vi "TLB Native Dynamic Events ver 0.04d.vi"() -> ()   [LabVIEW 2018]
uses:
  Labview Training Phase 2/Enum Controls/States for Action Engine.ctl
  Type def/TLB event states.ctl
  Type def/TLB MHL States.ctl
  <vilib>/Studica/Studica Toolkit/Background/I2C Channel.ctl
  <vilib>/Studica/Studica Toolkit/NavX/NavX.lvlib
  <vilib>/myRIO/Common/Instrument Driver Framework/myRIO v1.0/AI/typedefs/AI Channels Enum.ctl
  <vilib>/myRIO/Common/Instrument Driver Framework/myRIO v1.0/AI/typedefs/AI Channels List.ctl
  <vilib>/Studica/Studica Toolkit/Background/Mxp Selection.ctl
  <vilib>/ptbypt/NI_PtbyPt.lvlib
panel:
  out "Distance":T1
  in  "Return to IDLE":bool
  out "Sharp IR Distance":dbl
  out "Sharp IR Distance 2":dbl
  out "CM":fxp<+,64,16>
  out "Ultrasonic sensor":dbl format="%0.2f"
  out "Waveform Chart 3":dbl(graph)
  out "NavX Info Out":T3
  out "LinearAcceleration":T4
  out "Displacement":T5
  out "YRPHfH":T6
  in  "xTargetSpeed":dbl
  in  "yTargetSpeed":dbl
  in  "wTargetSpeed":dbl
  out "Speed":T7
  in  "Reset Encoder 0":bool
  out "Action Queue Items":i32
  out "State Logic Queue Items":i32
  out "Action Queues items":string[](array[string])=["Hardware reset", "Software reset", ""]
  out "State logic":T8=enum."Task 2"
  out "Action State":string
  in  "Tasks Selector":string(combo)="Task 2"
  in  "Stop Queue":bool
  in  "Start Task":bool
  # "Test Programme written by Calvin Loke    Dated: 28 Aug 2019\nTest Programme revised by Dr Alex See   Dated 30 Aug 2019\n\nProgramme version:   TLB Native Dynamic Events ver 0.04b.vi"
  # "System Health Status Update"
  # "Sequence of Actions"
  # "Continuous (Repeated)"
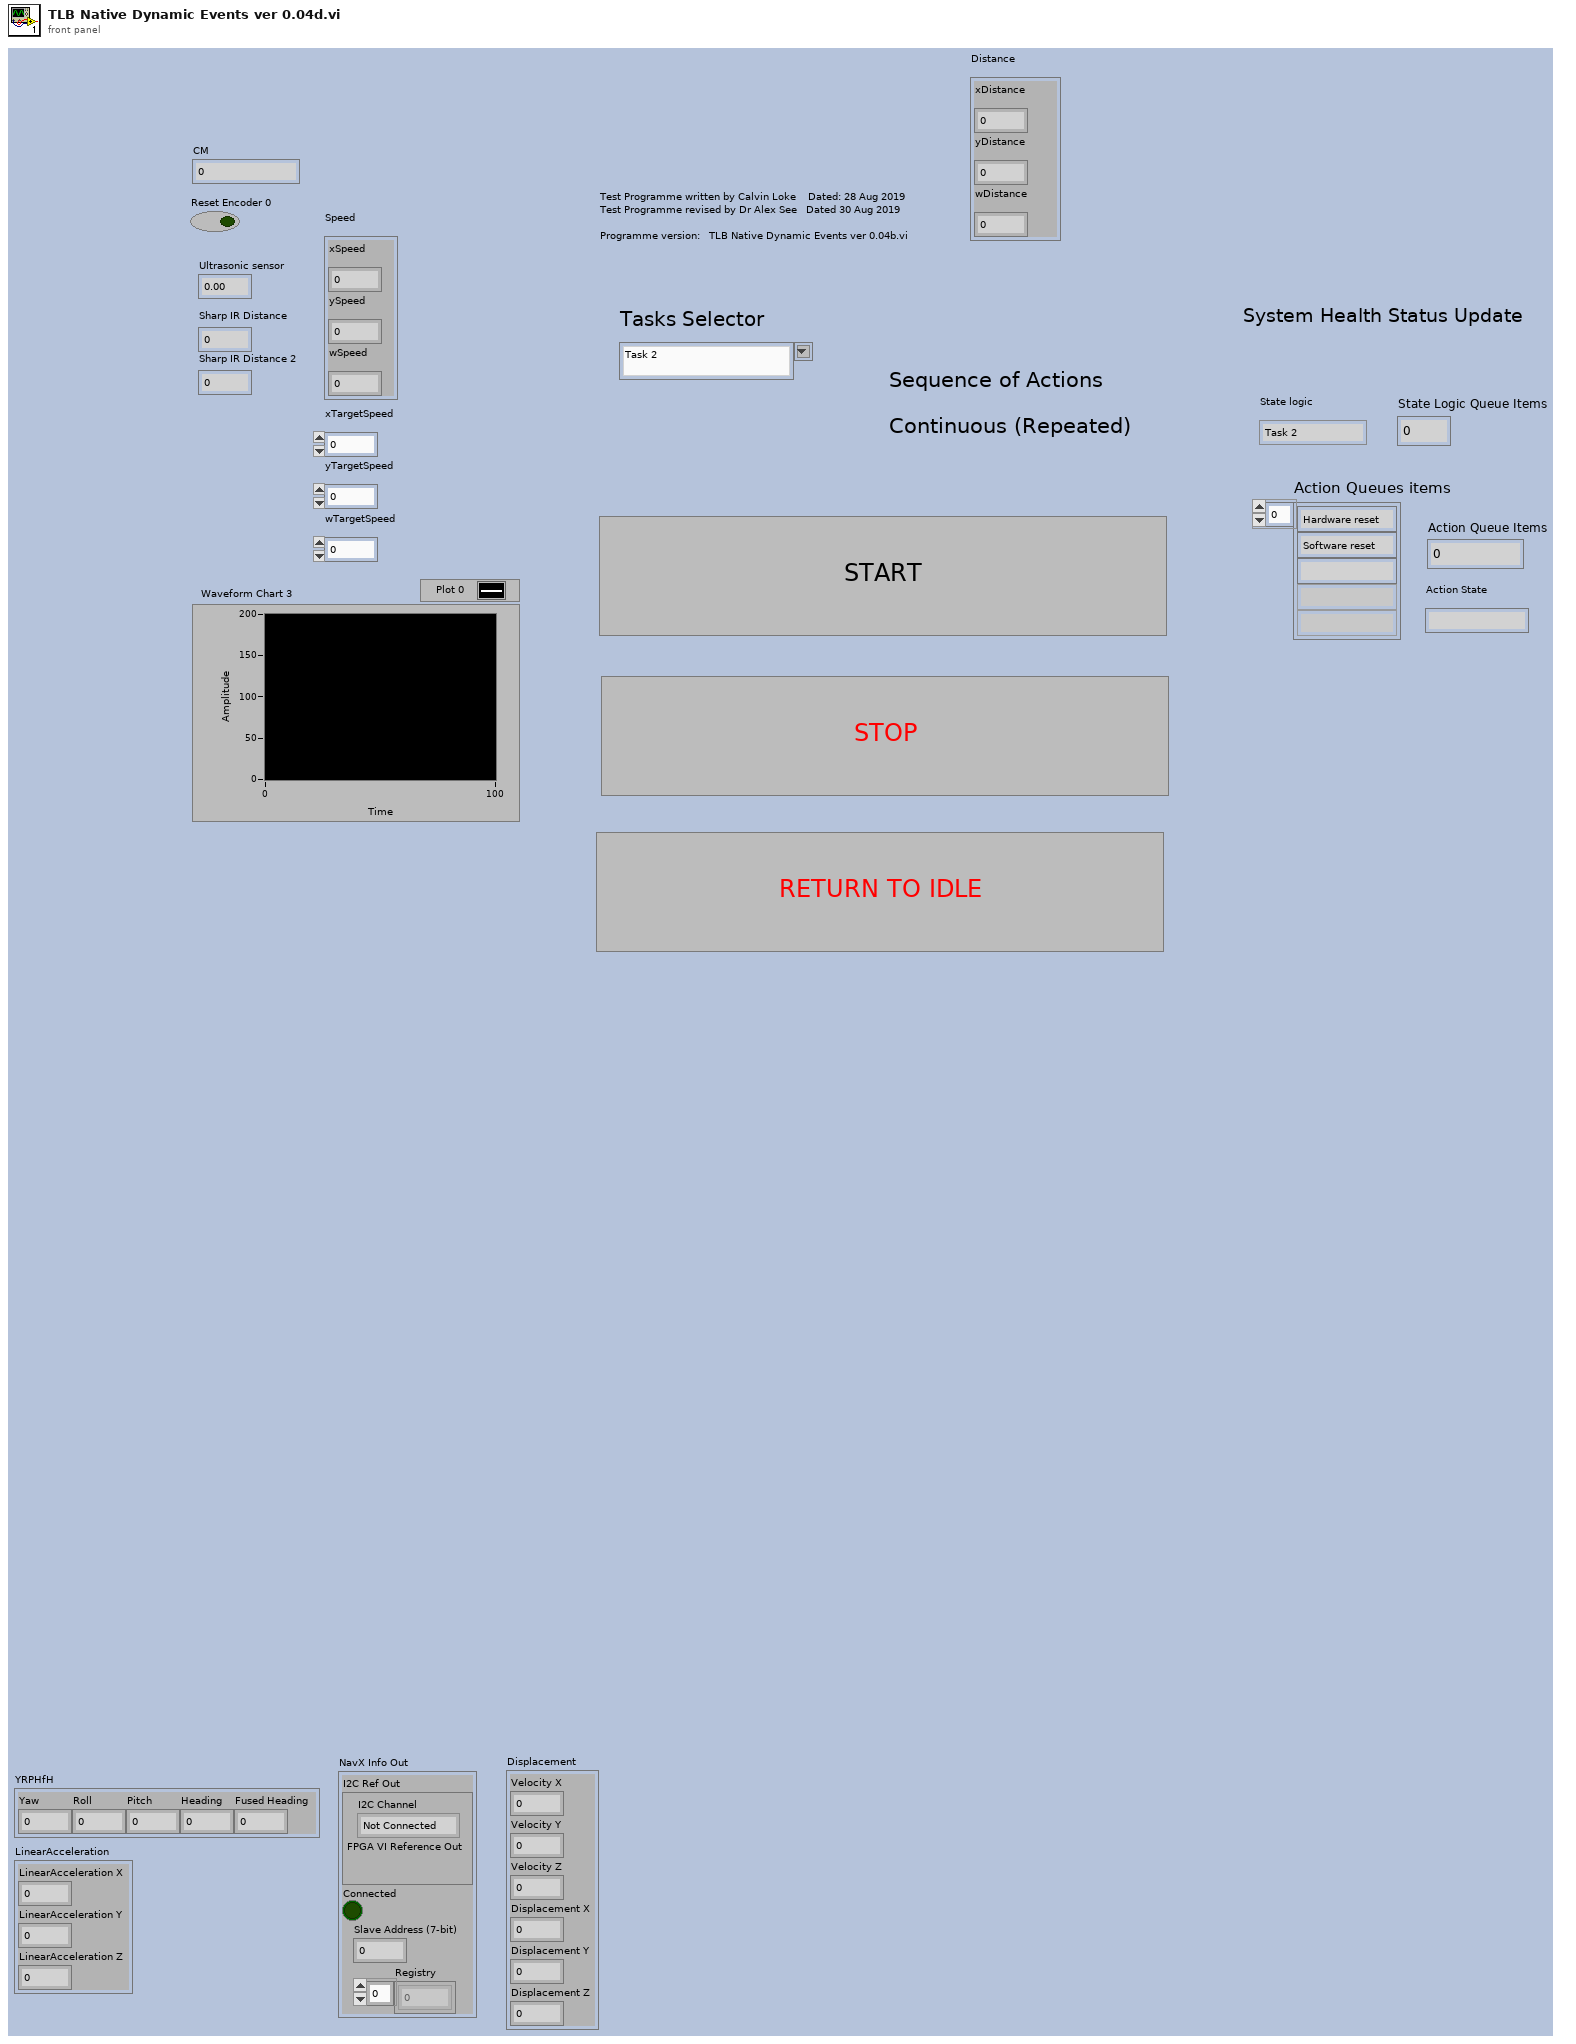
[diagram p1: front panel]
types:
  T1 = cluster{"xDistance":dbl, "yDistance":dbl, "wDistance":dbl}
  T2 = typedef "I2C Channel.ctl" = enum16{"Not Connected", "A", "B"}
  T3 = cluster{"I2C Ref Out":cluster{"I2C Channel":T2, "FPGA VI Reference Out":refnum<k20>}, "Connected":bool, "Slave Address (7-bit)":u8, "Registry":u8[]}
  T4 = cluster{"LinearAcceleration X":dbl, "LinearAcceleration Y":dbl, "LinearAcceleration Z":dbl}
  T5 = cluster{"Velocity X":dbl, "Velocity Y":dbl, "Velocity Z":dbl, "Displacement X":dbl, "Displacement Y":dbl, "Displacement Z":dbl}
  T6 = cluster{"Yaw":dbl, "Roll":dbl, "Pitch":dbl, "Heading":dbl, "Fused Heading":dbl}
  T7 = cluster{"xSpeed":dbl, "ySpeed":dbl, "wSpeed":dbl}
  T8 = typedef "TLB MHL States.ctl" = enum16{"None", "Startup", "Idle", "Processing", "Shutdown", "Reset", "Task 1", "Task 2", "Task 3", "Task 4", "Task 4a", "Task 4b", "Task 4c", "Task 4d", "Task 4e", "Task 4f", "Task 4g", "Task 4h", "Acquire image", "Wall follow mode", "Autodrive", "Autodrive a"}
  T9 = typedef "States for Action Engine.ctl" = enum16{"Initialize", "Write", "Read"}
  T10 = typedef "TLB event states.ctl" = enum16{"Start Sequence", "Exit", "Start Task 1", "Start Task 2", "Start Task 3", "Start Task 4", "Camera vision", "Wall follow mode", "Idle", "Start Drive Straight"}
  T11 = typedef "Mxp Selection.ctl" = enum16{"MXP A", "MXP B"}
  T12 = typedef "TLB event states.ctl" = enum16{"Start Sequence", "Exit", "Task 1", "Task 2", "Idle"}
  T13 = typedef "AI Channels List.ctl" = T14[]
  T14 = typedef "AI Channels Enum.ctl" = enum16{"Not Connected", "AudioIn/Left", "AudioIn/Right", "C/AI0", "C/AI1", "A/AI0", "A/AI1", "A/AI2", "A/AI3", "A/AI4", "A/AI5", "A/AI6", "A/AI7", "B/AI0", "B/AI1", "B/AI2", "B/AI3", "B/AI4", "B/AI5", "B/AI6", "B/AI7", "AI/AI0", "AI/AI1", "AI/AI2", "AI/AI3", "A/AI0 (DIFF)", "A/AI1 (DIFF)", "A/AI2 (DIFF)", "A/AI3 (DIFF)", "B/AI0 (DIFF)", "B/AI1 (DIFF)", "B/AI2 (DIFF)", "B/AI3 (DIFF)"}
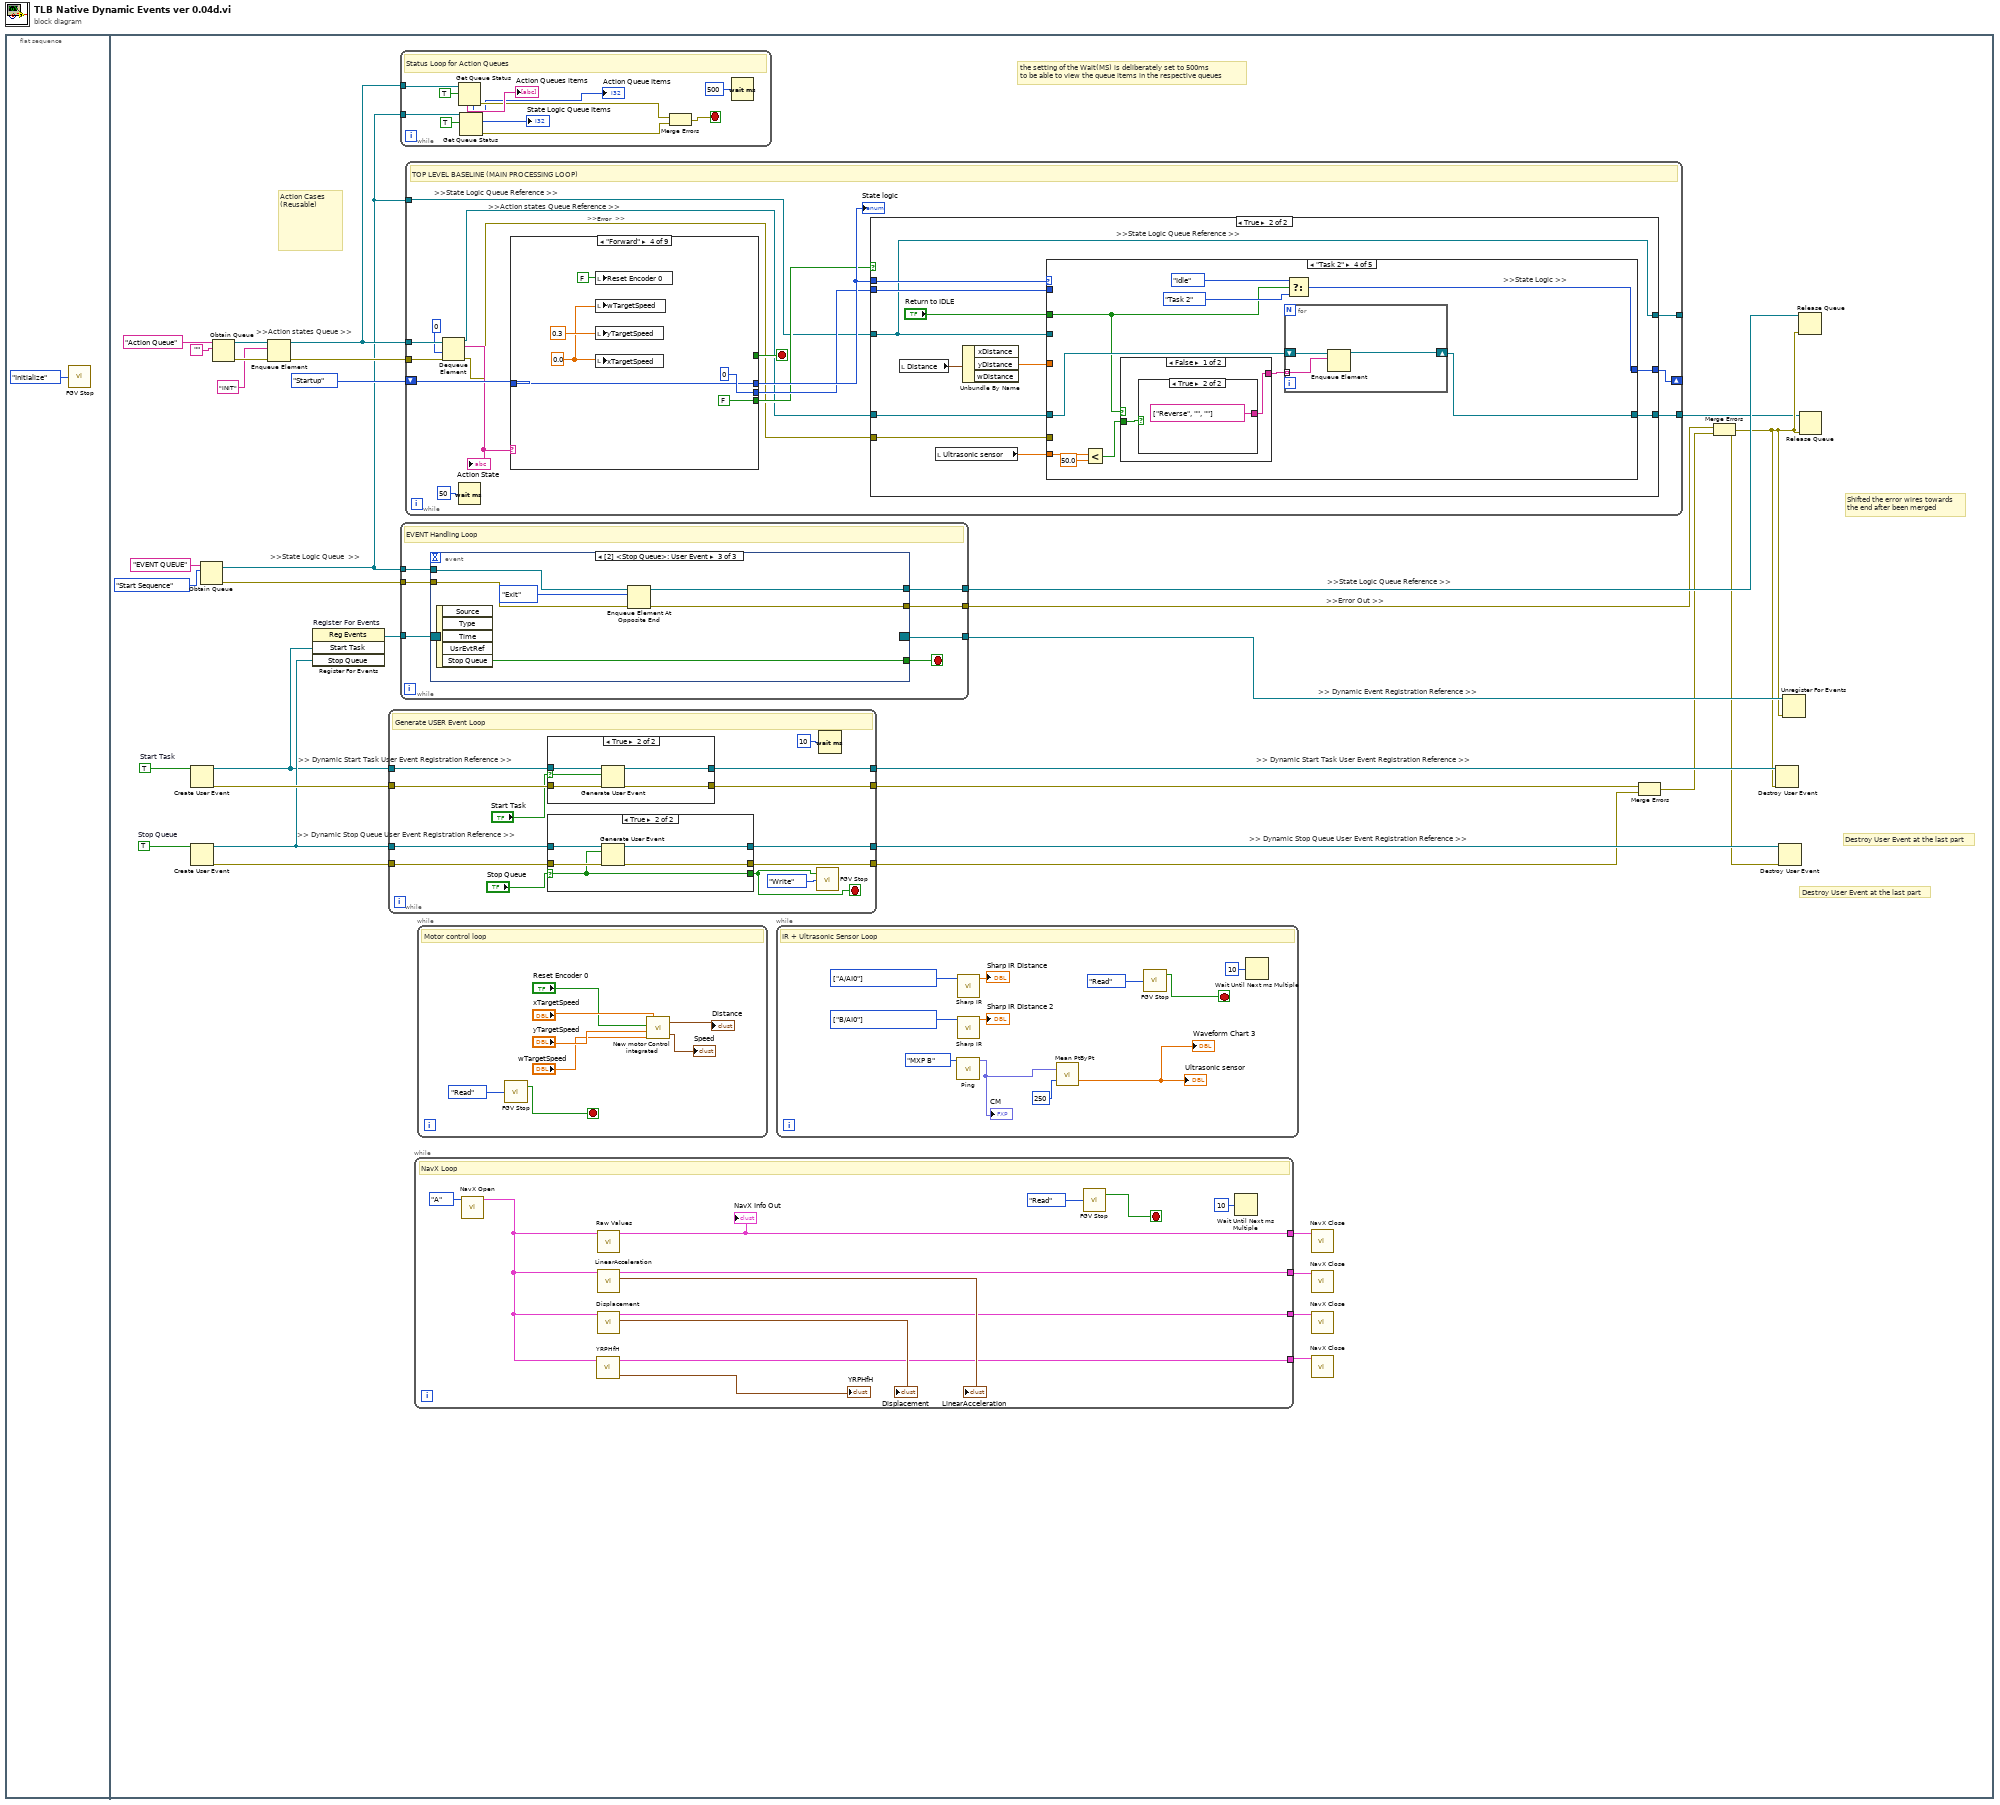
[diagram p0: block diagram]
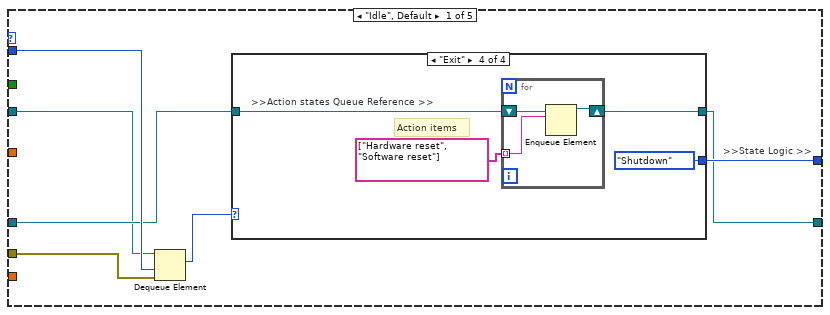
[diagram p3: hidden frame]
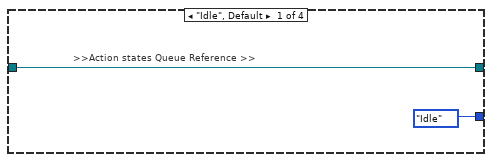
[diagram p4: hidden frame]
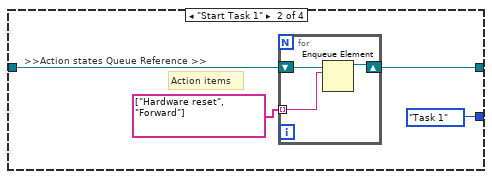
[diagram p5: hidden frame]
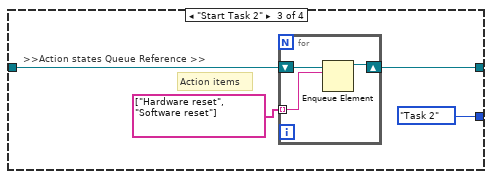
[diagram p6: hidden frame]
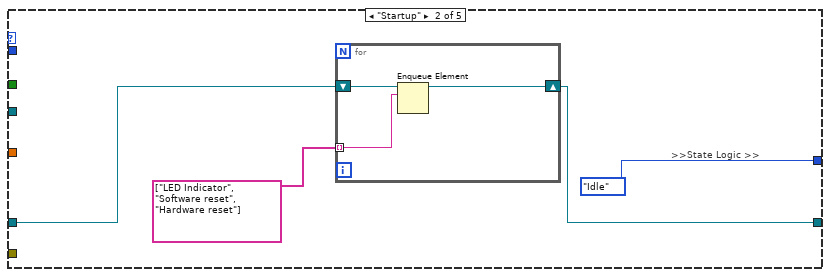
[diagram p7: hidden frame]
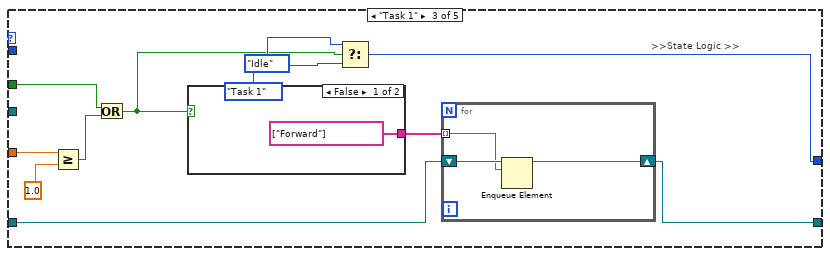
[diagram p8: hidden frame]
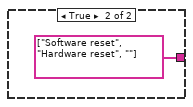
[diagram p9: hidden frame]
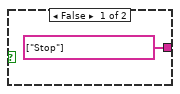
[diagram p10: hidden frame]
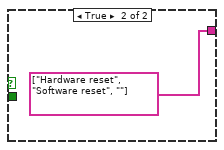
[diagram p11: hidden frame]
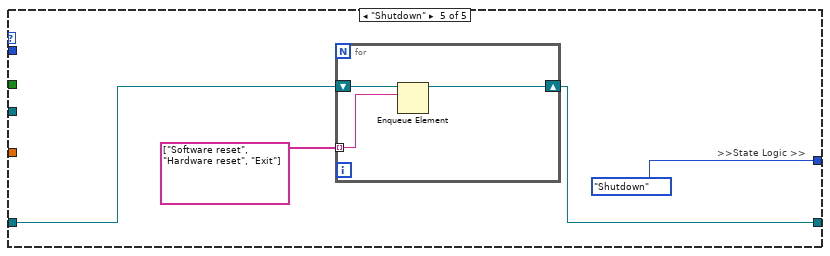
[diagram p12: hidden frame]
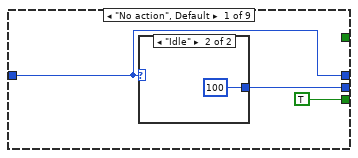
[diagram p13: hidden frame]
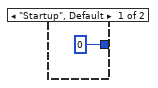
[diagram p14: hidden frame]
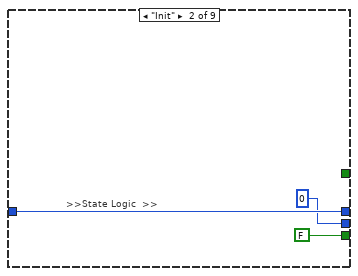
[diagram p15: hidden frame]
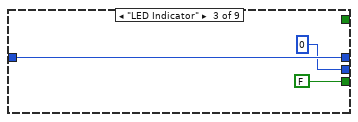
[diagram p16: hidden frame]
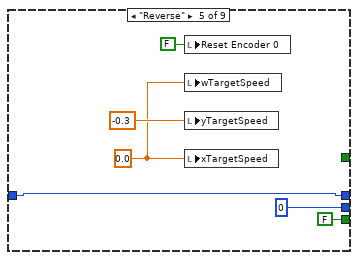
[diagram p17: hidden frame]
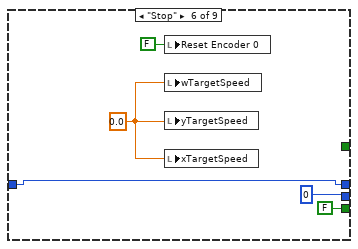
[diagram p18: hidden frame]
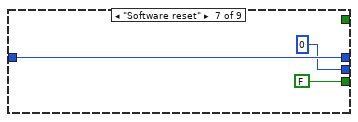
[diagram p19: hidden frame]
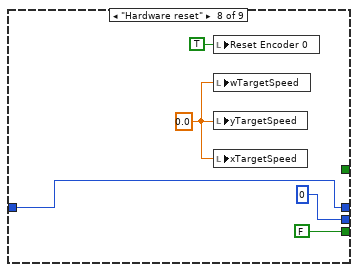
[diagram p20: hidden frame]
diagram:
  n1 = flat-sequence {
    frame #0 {
      n2 = call "FGV Stop.vi"("Init/Read/Write State"=States_for_Action_Engine."Initialize") -> ()  [unwired: 2 in, 2 out]
    }
    frame #1 {
      w34 = TRUE  # Stop Queue
      w33 = TRUE  # Start Task
      # "the setting of the Wait(MS) is deliberately set to 500ms\nto be able to view the queue items in the respective queues"
      # "Action Cases\n(Reusable)"
      # ">>Error Out >>"
      # ">> Dynamic Stop Queue User Event Registration Reference >>"
      # ">> Dynamic Start Task User Event Registration Reference >>"
      # ">> Dynamic Stop Queue User Event Registration Reference >>"
      # ">> Dynamic Start Task User Event Registration Reference >>"
      # ">> Dynamic Event Registration Reference >>"
      # ">>Action states Queue >>"
      # ">>State Logic Queue  >>"
      # ">>State Logic Queue Reference >>"
      # "Destroy User Event at the last part"
      # "Destroy User Event at the last part"
      # "Shifted the error wires towards\nthe end after been merged"
      n3 = Create User Event(user event datatype=w33) -> (user event=w25:refnum<user-event>, error out=w30:errorcluster)  [unwired: 1 in]
      n4 = Create User Event(user event datatype=w34) -> (user event=w26:refnum<user-event>, error out=w29:errorcluster)  [unwired: 1 in]
      n5 = Obtain Queue(name (unnamed)="EVENT QUEUE", element data type=TLB_event_states."Start Sequence" ("Enum")) -> (queue out=w9:refnum<queue>, error out=w15:errorcluster)  [unwired: 3 in, 1 out]
      n6 = Obtain Queue(name (unnamed)="Action Queue", element data type="") -> (queue out=w18:refnum<queue>, error out=w14:errorcluster)  [unwired: 3 in, 1 out]
      n7 = Enqueue Element(queue=w18, element="INIT", error in (no error)=w14) -> (queue out=w10:refnum<queue>, error out=w13:errorcluster)  [unwired: 1 in, 1 out]
      n8 = register-events "Register For Events"(w25, w26) -> (reference out=w24:refnum<event-registration>)  [unwired: 2 in, 1 out]
      n9 = while {
        tunnel: w25 -> [w265]
        tunnel: w26 -> [w264]
        tunnel: [w263] -> w32
        tunnel: [w262] -> w31
        tunnel: w30 -> [w261]
        tunnel: [w260] -> w28
        tunnel: w29 -> [w259]
        tunnel: [w258] -> w27
        stop <- w254 stop-if-true
        # "Generate USER Event Loop"
        n10 = case shown="True" "Start Task" {
          selector: "Start Task" -> [_ w277]
          tunnel: w265 -> [w276 w281]
          tunnel: [w276 w280] -> w262
          tunnel: w261 -> [w275 w279]
          tunnel: [w275 w278] -> w260
          frame False {
          }
          frame True {
            n11 = Generate User Event(user event=w281, event data cluster=w277, error in=w279) -> (user event out=w280:refnum<user-event>, error out=w278:errorcluster)  [unwired: 1 in]
          }
        }
        n12 = case shown="True" "Stop Queue" {
          selector: "Stop Queue" -> [_ w270]
          tunnel: w264 -> [w269 w274]
          tunnel: [w269 w273] -> w263
          tunnel: w259 -> [w268 w272]
          tunnel: [w268 w271] -> w258
          tunnel: [FALSE w270] -> w254
          frame False {
          }
          frame True {
            n13 = Generate User Event(user event=w274, event data cluster=w270, error in=w272) -> (user event out=w273:refnum<user-event>, error out=w271:errorcluster)  [unwired: 1 in]
          }
        }
        n14 = call "FGV Stop.vi"("Init/Read/Write State"=States_for_Action_Engine."Write", "Input Node"=w254) -> ()  [unwired: 1 in, 2 out]
        n15 = Wait (ms)(milliseconds to wait=u32 10) -> ()  [unwired: 1 out]
      }
      n16 = while {
        tunnel: w10 -> [w74]
        tunnel: w9 -> [w71]
        stop <- w68 stop-if-true
        # "Status Loop for Action Queues"
        n17 = Get Queue Status(queue=w74, return elements? (F)=TRUE) -> (error out=w70:errorcluster, # elements in queue=→"Action Queue Items":i32, elements=→"Action Queues items":string[])  [unwired: 1 in, 5 out]
        n18 = Get Queue Status(queue=w71, return elements? (F)=TRUE) -> (# pending remove=→"State Logic Queue Items":i32, error out=w69:errorcluster)  [unwired: 1 in, 6 out]
        n19 = Merge Errors(w70, w69) -> (w68:errorcluster)
        n20 = Wait (ms)(milliseconds to wait=u32 500) -> ()  [unwired: 1 out]
      }
      n21 = while {
        tunnel: w24 -> [w231]
        tunnel: [w230] -> w23
        tunnel: w9 -> [w228]
        tunnel: [w227] -> w22
        tunnel: w15 -> [w226]
        tunnel: [w225] -> w12
        stop <- w229 stop-if-true
        # "EVENT Handling Loop"
        n22 = event shown="[2] <Stop Queue>: User Event" {
          selector: w231 -> [_ _ _]
          dyn-events: [_ _ _] -> w230
          timeout: _ -> [_ _ _]
          tunnel: [FALSE FALSE w253] -> w229
          tunnel: w228 -> [w236 w243 w251]
          tunnel: [w235 w242 w252] -> w227
          tunnel: w226 -> [w233 w239 w249]
          tunnel: [w232 w238 w248] -> w225
          event Timeout {
            n23 = event-data() -> ()  [unwired: 1 in, 3 out]
            n24 = Enqueue Element(queue=w236, element=TLB_event_states."Idle" ("Enum"), error in (no error)=w233) -> (queue out=w235:refnum<queue>, error out=w232:errorcluster)  [unwired: 1 in, 1 out]
          }
          event User Event {
            n25 = event-data() -> ()  [unwired: 1 in, 5 out]
            n26 = case shown="Default" "Tasks Selector" {
              tunnel: [TLB_event_states."Idle" ("Enum") TLB_event_states."Start Task 1" ("Enum") TLB_event_states."Task 2" ("Enum")] -> w240
              frame Default {
              }
              frame "Task 1" {
              }
              frame "Task 2" {
              }
            }
            n27 = Enqueue Element(queue=w243, element=w240, error in (no error)=w239) -> (queue out=w242:refnum<queue>, error out=w238:errorcluster)  [unwired: 1 in, 1 out]
          }
          event User Event {
            n28 = event-data() -> ("Stop Queue"=w253:bool)  [unwired: 1 in, 4 out]
            n29 = Enqueue Element At Opposite End(queue=w251, element=TLB_event_states."Exit" ("Enum"), error in (no error)=w249) -> (queue out=w252:refnum<queue>, error out=w248:errorcluster)  [unwired: 1 in, 1 out]
          }
        }
      }
      n30 = while {
        tunnel: w9 -> [w79]
        shift-right: [w84] -> _
        shift-left: TLB_MHL_States."Startup" ("Enum") -> [w91]
        tunnel: w10 -> [w89]
        tunnel: w13 -> [w87]
        tunnel: [w86] -> _
        tunnel: [w85] -> w7
        stop <- w82 stop-if-true
        # ">>Error  >>"
        # ">>Action states Queue Reference >>"
        # ">>State Logic Queue Reference >>"
        # "TOP LEVEL BASELINE (MAIN PROCESSING LOOP)"
        n31 = Dequeue Element(queue=w89, timeout in ms (-1)=0, error in (no error)=w87) -> (queue out=w78:refnum<queue>, element=w88:string, error out=w77:errorcluster)  [unwired: 1 out]
        "Action State" <- w88
        n32 = Wait (ms)(milliseconds to wait=u32 50) -> ()  [unwired: 1 out]
        n33 = case shown="\"Forward\"" w88 {
          tunnel: [w187 w192 w195 w200 w206 w211 w215 w220 TLB_MHL_States."Shutdown" ("Enum")] -> w90
          tunnel: w91 -> [w187 w192 w195 w200 w206 w211 w215 w220 _]
          tunnel: [w186 0 0 0 0 0 0 0 0] -> w83
          tunnel: [_ _ _ _ _ _ _ _ TRUE] -> w82
          tunnel: [TRUE FALSE FALSE FALSE FALSE FALSE FALSE FALSE FALSE] -> w81
          frame "No action", Default {
            n34 = case shown="\"Idle\"" w187 {
              tunnel: [0 100] -> w186
              frame "Startup", Default {
              }
              frame "Idle" {
              }
            }
          }
          frame "Init" {
            # ">>State Logic  >>"
          }
          frame "LED Indicator" {
          }
          frame "Forward" {
            w196 = 0.0
            n35 = local write "Reset Encoder 0"(FALSE ("Reset Encoder 0")) -> ()
            n36 = local write "wTargetSpeed"(w196) -> ()
            n37 = local write "yTargetSpeed"(0.3 ("yTargetSpeed")) -> ()
            n38 = local write "xTargetSpeed"(w196) -> ()
          }
          frame "Reverse" {
            w202 = 0.0
            n39 = local write "Reset Encoder 0"(FALSE ("Reset Encoder 0")) -> ()
            n40 = local write "wTargetSpeed"(w202) -> ()
            n41 = local write "yTargetSpeed"(-0.3 ("yTargetSpeed")) -> ()
            n42 = local write "xTargetSpeed"(w202) -> ()
          }
          frame "Stop" {
            w208 = 0.0
            n43 = local write "Reset Encoder 0"(FALSE ("Reset Encoder 0")) -> ()
            n44 = local write "wTargetSpeed"(w208) -> ()
            n45 = local write "yTargetSpeed"(w208) -> ()
            n46 = local write "xTargetSpeed"(w208) -> ()
          }
          frame "Software reset" {
          }
          frame "Hardware reset" {
            w216 = 0.0
            n47 = local write "Reset Encoder 0"(TRUE ("Reset Encoder 0")) -> ()
            n48 = local write "wTargetSpeed"(w216) -> ()
            n49 = local write "yTargetSpeed"(w216) -> ()
            n50 = local write "xTargetSpeed"(w216) -> ()
          }
          frame "Exit" {
          }
        }
        "State logic" <- w90
        n51 = case shown="True" w81 {
          tunnel: w90 -> [w94 w106]
          tunnel: w79 -> [w95 w100]
          tunnel: w78 -> [w93 w105]
          tunnel: [w95 w100] -> w86
          tunnel: [w93 w104] -> w85
          tunnel: [w94 w103] -> w84
          tunnel: w77 -> [_ w102]
          tunnel: w83 -> [_ w101]
          frame False {
          }
          frame True {
            # ">>State Logic Queue Reference >>"
            n52 = local read "Distance"() -> (w98:T1)
            n53 = local read "Ultrasonic sensor"() -> (w96:dbl)
            n54 = Unbundle By Name(w98) -> ("yDistance"=w97:dbl)  [unwired: 2 out]
            n55 = case shown="\"Task 2\"" w106 {
              tunnel: w100 -> [w107 _ _ _ _]
              tunnel: w105 -> [w109 w138 w150 w165 w179]
              tunnel: [w108 w137 w149 w166 w178] -> w104
              tunnel: [w112 TLB_MHL_States."Idle" ("Enum") w152 w167 TLB_MHL_States."Shutdown" ("Enum")] -> w103
              tunnel: w102 -> [w110 _ _ _ _]
              tunnel: w101 -> [w111 _ _ _ _]
              tunnel: "Return to IDLE" -> [_ _ w147 w162 _]
              tunnel: w97 -> [_ _ w146 _ _]
              tunnel: w96 -> [_ _ _ w164 _]
              frame "Idle", Default {
                # ">>State Logic >>"
                n56 = Dequeue Element(queue=w107, timeout in ms (-1)=w111, error in (no error)=w110) -> (element=w113:T10)  [unwired: 3 out]
                n57 = case shown="\"Exit\"" w113 {
                  tunnel: [TLB_MHL_States."Idle" ("Enum") TLB_MHL_States."Task 1" ("Enum") TLB_MHL_States."Task 2" ("Enum") TLB_MHL_States."Shutdown" ("Enum")] -> w112
                  tunnel: [w114 w118 w123 w130] -> w108
                  tunnel: w109 -> [w114 w116 w124 w131]
                  frame "Idle", Default {
                    # ">>Action states Queue Reference >>"
                  }
                  frame "Start Task 1" {
                    # ">>Action states Queue Reference >>"
                    # "Action items"
                    n58 = for {
                      shift-right: [w122] -> w118
                      shift-left: w116 -> [w121]
                      tunnel: string[] ["Hardware reset", "Forward"] -> [w120] mode=indexing
                      n59 = Enqueue Element(queue=w121, element=w120) -> (queue out=w122:refnum<queue>)  [unwired: 2 in, 2 out]
                    }
                  }
                  frame "Start Task 2" {
                    # ">>Action states Queue Reference >>"
                    # "Action items"
                    n60 = for {
                      shift-right: [w129] -> w123
                      shift-left: w124 -> [w128]
                      tunnel: string[] ["Hardware reset", "Software reset"] -> [w127] mode=indexing
                      n61 = Enqueue Element(queue=w128, element=w127) -> (queue out=w129:refnum<queue>)  [unwired: 2 in, 2 out]
                    }
                  }
                  frame "Exit" {
                    # ">>Action states Queue Reference >>"
                    # "Action items"
                    n62 = for {
                      shift-right: [w136] -> w130
                      shift-left: w131 -> [w135]
                      tunnel: string[] ["Hardware reset", "Software reset"] -> [w134] mode=indexing
                      n63 = Enqueue Element(queue=w135, element=w134) -> (queue out=w136:refnum<queue>)  [unwired: 2 in, 2 out]
                    }
                  }
                }
              }
              frame "Startup" {
                # ">>State Logic >>"
                n64 = for {
                  shift-right: [w142] -> w137
                  shift-left: w138 -> [w143]
                  tunnel: string[] ["LED Indicator", "Software reset", "Hardware reset"] -> [w141] mode=indexing
                  n65 = Enqueue Element(queue=w143, element=w141) -> (queue out=w142:refnum<queue>)  [unwired: 2 in, 2 out]
                }
              }
              frame "Task 1" {
                # ">>State Logic >>"
                n66 = Greater Or Equal?(x=w146, y=1.0) -> (x >= y?=w144:bool)
                n67 = Or(x=w147, y=w144) -> (x .or. y?=w148:bool)
                n68 = case shown="False" w148 {
                  tunnel: [string[] ["Forward"] string[] ["Software reset", "Hardware reset", ""]] -> w151
                  frame False {
                  }
                  frame True {
                  }
                }
                n69 = Select(t=TLB_MHL_States."Idle" ("Enum"), s=w148, f=TLB_MHL_States."Task 1" ("Enum")) -> (s? t:f=w152:T8)
                n70 = for {
                  shift-right: [w158] -> w149
                  shift-left: w150 -> [w159]
                  tunnel: w151 -> [w157] mode=indexing
                  n71 = Enqueue Element(queue=w159, element=w157) -> (queue out=w158:refnum<queue>)  [unwired: 2 in, 2 out]
                }
              }
              frame "Task 2" {
                # ">>State Logic >>"
                n72 = Less?(x=w164, y=50.0) -> (x < y?=w160:bool)
                n73 = case shown="False" w162 {
                  tunnel: [w170 string[] ["Hardware reset", "Software reset", ""]] -> w161
                  tunnel: w160 -> [w171 _]
                  frame False {
                    n74 = case shown="True" w171 {
                      tunnel: [string[] ["Stop"] string[] ["Reverse", "", ""]] -> w170
                      frame False {
                      }
                      frame True {
                      }
                    }
                  }
                  frame True {
                  }
                }
                n75 = for {
                  shift-right: [w176] -> w166
                  shift-left: w165 -> [w177]
                  tunnel: w161 -> [w175] mode=indexing
                  n76 = Enqueue Element(queue=w177, element=w175) -> (queue out=w176:refnum<queue>)  [unwired: 2 in, 2 out]
                }
                n77 = Select(t=TLB_MHL_States."Idle" ("Enum"), s=w162, f=TLB_MHL_States."Task 2" ("Enum")) -> (s? t:f=w167:T8)
              }
              frame "Shutdown" {
                # ">>State Logic >>"
                n78 = for {
                  shift-right: [w183] -> w178
                  shift-left: w179 -> [w184]
                  tunnel: string[] ["Software reset", "Hardware reset", "Exit"] -> [w182] mode=indexing
                  n79 = Enqueue Element(queue=w184, element=w182) -> (queue out=w183:refnum<queue>)  [unwired: 2 in, 2 out]
                }
              }
            }
          }
        }
      }
      n80 = while {
        tunnel: [w54] -> w5
        tunnel: [w50] -> w4
        tunnel: [w49] -> w2
        tunnel: [w48] -> w3
        stop <- w56 stop-if-true
        # "NavX Loop"
        n81 = call <vilib>:"NavX Open.vi"("I2C Channel"=I2C_Channel."A") -> ("NavX Info"=w46:T3)  [unwired: 9 in, 1 out]
        n82 = call <vilib>:"YRPHfH.vi"("NavX Info In"=w46) -> ("YRPHfH"=→"YRPHfH":T6, "NavX Info Out"=w49:T3)  [unwired: 3 in]
        n83 = call <vilib>:"Raw Values.vi"("NavX Info In"=w46) -> ("NavX Info Out"=w54:T3)  [unwired: 8 in, 1 out]
        "NavX Info Out" <- w54
        n84 = call <vilib>:"LinearAcceleration.vi"("NavX Info In"=w46) -> ("LinearAcceleration"=→"LinearAcceleration":T4, "NavX Info Out"=w50:T3)  [unwired: 9 in]
        n85 = call <vilib>:"Displacement.vi"("NavX Info In"=w46) -> ("Displacement"=→"Displacement":T5, "NavX Info Out"=w48:T3)  [unwired: 9 in]
        n86 = call "FGV Stop.vi"("Init/Read/Write State"=States_for_Action_Engine."Read") -> ("Output node"=w56:bool)  [unwired: 2 in, 1 out]
        n87 = Wait Until Next ms Multiple(millisecond multiple=u32 10) -> ()  [unwired: 1 out]
      }
      n88 = while {
        stop <- w64 stop-if-true
        # "Motor control loop"
        n89 = call "FGV Stop.vi"("Init/Read/Write State"=States_for_Action_Engine."Read") -> ("Output node"=w64:bool)  [unwired: 2 in, 1 out]
        n90 = call "New motor Control integrated.vi"("wTargetSpeed"="wTargetSpeed", "yTargetSpeed"="yTargetSpeed", "xTargetSpeed"="Reset Encoder 0", "Reset Encoders"="xTargetSpeed") -> ("Speed"=→"Speed":T7, "Distance"=→"Distance":T1)
      }
      n91 = while {
        stop <- w39 stop-if-true
        w44 = T13 [enum."B/AI0"] items=["Not Connected", "AudioIn/Left", "AudioIn/Right", "C/AI0", "C/AI1", "A/AI0", "A/AI1", "A/AI2", "A/AI3", "A/AI4", "A/AI5", "A/AI6", "A/AI7", "B/AI0", "B/AI1", "B/AI2", "B/AI3", "B/AI4", "B/AI5", "B/AI6", "B/AI7", "AI/AI0", "AI/AI1", "AI/AI2", "AI/AI3", "A/AI0 (DIFF)", "A/AI1 (DIFF)", "A/AI2 (DIFF)", "A/AI3 (DIFF)", "B/AI0 (DIFF)", "B/AI1 (DIFF)", "B/AI2 (DIFF)", "B/AI3 (DIFF)"] ("AI Channel")
        w45 = T13 [enum."A/AI0"] items=["Not Connected", "AudioIn/Left", "AudioIn/Right", "C/AI0", "C/AI1", "A/AI0", "A/AI1", "A/AI2", "A/AI3", "A/AI4", "A/AI5", "A/AI6", "A/AI7", "B/AI0", "B/AI1", "B/AI2", "B/AI3", "B/AI4", "B/AI5", "B/AI6", "B/AI7", "AI/AI0", "AI/AI1", "AI/AI2", "AI/AI3", "A/AI0 (DIFF)", "A/AI1 (DIFF)", "A/AI2 (DIFF)", "A/AI3 (DIFF)", "B/AI0 (DIFF)", "B/AI1 (DIFF)", "B/AI2 (DIFF)", "B/AI3 (DIFF)"] ("AI Channel")
        # "IR + Ultrasonic Sensor Loop"
        n92 = call <vilib>:"Ping.vi"("Mxp Side"=Mxp_Selection."MXP B") -> ("CM"=w35:fxp<+,64,16>)  [unwired: 8 in, 2 out]
        "CM" <- w35
        n93 = call <vilib>:"Sharp IR.vi"("AI Channel"=w45) -> ("Sharp IR Distance"=→"Sharp IR Distance":dbl)  [unwired: 8 in, 2 out]
        n94 = call <vilib>:"Sharp IR.vi"("AI Channel"=w44) -> ("Sharp IR Distance"=→"Sharp IR Distance 2":dbl)  [unwired: 8 in, 2 out]
        n95 = call <vilib>:"Mean PtByPt.vi"("x"=w35, "sample length"=250) -> ("mean"=→"Ultrasonic sensor" →"Waveform Chart 3":dbl)  [unwired: 2 in, 1 out]
        n96 = call "FGV Stop.vi"("Init/Read/Write State"=States_for_Action_Engine."Read") -> ("Output node"=w39:bool)  [unwired: 2 in, 1 out]
        n97 = Wait Until Next ms Multiple(millisecond multiple=u32 10) -> ()  [unwired: 1 out]
      }
      n98 = call <vilib>:"NavX Close.vi"("NavX Info In"=w5) -> ()  [unwired: 10 in, 1 out]
      n99 = call <vilib>:"NavX Close.vi"("NavX Info In"=w4) -> ()  [unwired: 10 in, 1 out]
      n100 = call <vilib>:"NavX Close.vi"("NavX Info In"=w3) -> ()  [unwired: 10 in, 1 out]
      n101 = call <vilib>:"NavX Close.vi"("NavX Info In"=w2) -> ()  [unwired: 10 in, 1 out]
      n102 = Merge Errors "Merge Errors"(w28, w27) -> (w6:errorcluster)
      n103 = Merge Errors(w12, w6) -> (w8:errorcluster)
      n104 = Destroy User Event(user event=w31, error in=w8) -> ()  [unwired: 1 out]
      n105 = Destroy User Event(user event=w32, error in=w8) -> ()  [unwired: 1 out]
      n106 = Unregister For Events(event registration refnum=w23, error in=w8) -> ()  [unwired: 1 out]
      n107 = Release Queue(queue=w22, error in (no error)=w8) -> ()  [unwired: 1 in, 3 out]
      n108 = Release Queue(queue=w7, error in (no error)=w8) -> ()  [unwired: 1 in, 3 out]
    }
  }
